vi "Get Current Branch Name.vi"(8 "error in":errorcluster, 11 "Peer Review in":refnum<class "Peer Review.lvclass">) -> (0 "error out":errorcluster, 3 "Peer Review out":refnum<class "Peer Review.lvclass">)   [LabVIEW 2020, in "Peer Review.lvclass"]
uses:
  Peer Review.lvclass
  Peer Review.lvclass/Peer Review.ctl
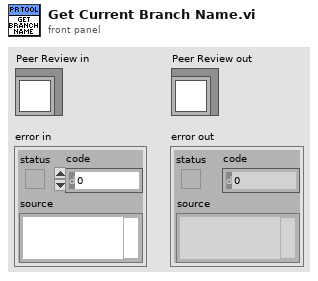
[diagram p1: front panel]
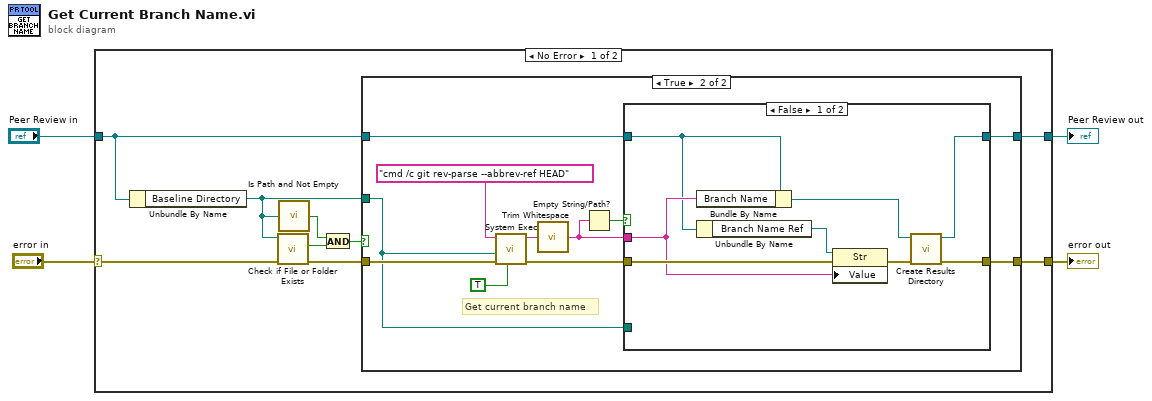
[diagram p0: block diagram]
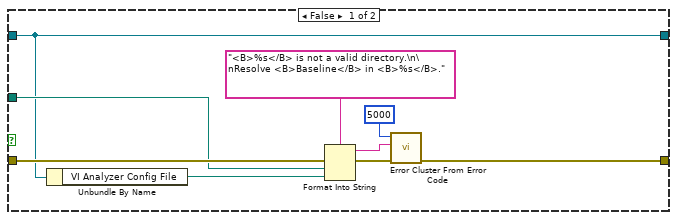
[diagram p2: hidden frame]
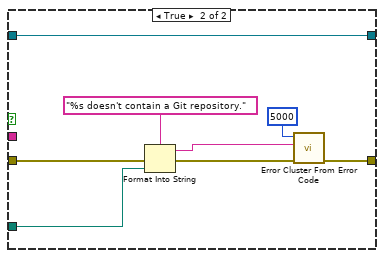
[diagram p3: hidden frame]
diagram:
  n1 = case shown="No Error" "error in" {
    selector: "error in" -> [w10 w51]
    tunnel: [w12 w51] -> w3
    tunnel: [w11 w50] -> w1
    tunnel: "Peer Review in" -> [w13 w50]
    frame No Error {
      n2 = Unbundle By Name(w13) -> ("Baseline Directory"=w8:path)
      n3 = call <vilib>:"Check if File or Folder Exists.vi"("error in (no error)"=w10, "path"=w8) -> ("error out"=w9:errorcluster, "file or folder exists?"=w7:bool)  [unwired: 7 in, 1 out]
      n4 = call <vilib>:"Is Path and Not Empty.vi"("path"=w8) -> ("Is Path and Not Empty?"=w6:bool)  [unwired: 4 in]
      n5 = And(x=w6, y=w7) -> (x .and. y?=w5:bool)
      n6 = case shown="True" w5 {
        tunnel: w13 -> [w15 w23]
        tunnel: [w17 w29] -> w12
        tunnel: [w15 w28] -> w11
        tunnel: w9 -> [w18 w26]
        tunnel: w8 -> [w16 w25]
        frame False {
          n7 = Unbundle By Name(w15) -> ("VI Analyzer Config File"=w14:path)
          n8 = Format Into String(format string="<B>%s</B> is not a valid directory.\n\nResolve <B>Baseline</B> in <B>%s</B>." ("error message (\"\")"), error in=w18, w16, w14) -> (resulting string=w19:string, error out=w21:errorcluster)  [unwired: 1 in]
          n9 = call <vilib>:"Error Cluster From Error Code.vi"("error in (no error)"=w21, "error message (\"\")"=w19, "error code (0)"=5000) -> ("error out"=w17:errorcluster)  [unwired: 6 in]
        }
        frame True {
          # "Get current branch name"
          n10 = call <vilib>:"System Exec.vi"("run minimized? (F)"=TRUE, "error in (no error)"=w26, "working directory"=w25, "command line"="cmd /c git rev-parse --abbrev-ref HEAD" ("String 2")) -> ("error out"=w30:errorcluster, "standard output"=w33:string)  [unwired: 4 in, 2 out]
          n11 = call <vilib>:"Trim Whitespace.vi"("string"=w33) -> ("trimmed string"=w27:string)  [unwired: 1 in]
          n12 = Empty String/Path?(string/path=w27) -> (empty?=w24:bool)
          n13 = case shown="False" w24 {
            tunnel: w23 -> [w35 w42]
            tunnel: w30 -> [w41 w48]
            tunnel: [w39 w45] -> w29
            tunnel: [w37 w42] -> w28
            tunnel: w27 -> [w36 _]
            tunnel: w25 -> [_ w47]
            frame False {
              n14 = Bundle By Name(cluster=w35, "Branch Name"=w36) -> (w38:refnum<class "Peer Review.lvclass">)
              n15 = Unbundle By Name(w35) -> ("Branch Name Ref"=w34:refnum<vi>)
              n16 = property class="Str"(reference=w34, error in=w41, "Value"=w36) -> (error out=w40:errorcluster)  [unwired: 1 out]
              n17 = call "Create Results Directory.vi"("error in"=w40, "Peer Review in"=w38) -> ("error out"=w39:errorcluster, "Peer Review out"=w37:refnum<class "Peer Review.lvclass">)  [unwired: 8 in]
            }
            frame True {
              n18 = Format Into String(format string="%s doesn't contain a Git repository." ("error message (\"\")"), error in=w48, w47) -> (resulting string=w44:string, error out=w49:errorcluster)  [unwired: 1 in]
              n19 = call <vilib>:"Error Cluster From Error Code.vi"("error in (no error)"=w49, "error message (\"\")"=w44, "error code (0)"=5000) -> ("error out"=w45:errorcluster)  [unwired: 6 in]
            }
          }
        }
      }
    }
    frame Error {
    }
  }
  "error out" <- w3
  "Peer Review out" <- w1
